vi "white line 1.vi"   [LabVIEW 2010, in "Line Follower.lvrbt"]
uses:
  Line Follower.lvrbt
  <vilib>/NXT/Block Support/NXT_InputPort.ctl
  <vilib>/NXT/Subs/MotorOutput.ctl
  <vilib>/NXT/Dual Mode Library/Sensors/Sonar_cm.vi
  <vilib>/NXT/Dual Mode Library/Sensors/Light_On.vi
  <vilib>/NXT/Dual Mode Library/Motors/MotorOn.vi
  <vilib>/NXT/Dual Mode Library/Motors/MotorBrake.vi
types:
  T1 = typedef "NXT_InputPort.ctl" = u8
  T2 = typedef "MotorOutput.ctl" = u8
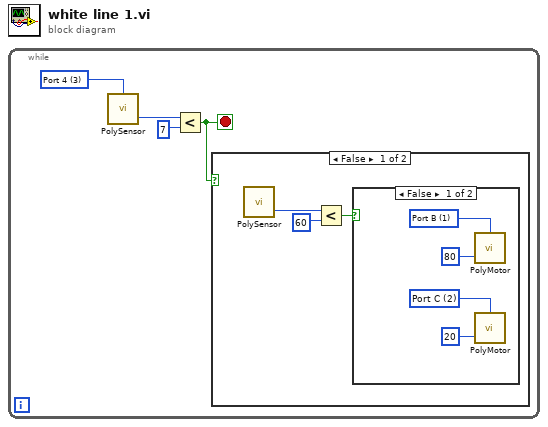
[diagram p0: block diagram]
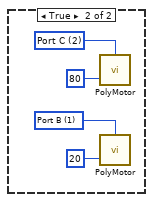
[diagram p2: hidden frame]
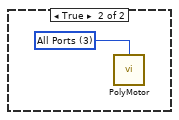
[diagram p3: hidden frame]
diagram:
  n1 = while {
    stop <- w2 stop-if-true
    w4 = T1 3 items=["Port 1", "Port 2", "Port 3", "Port 4"] ("Port (Port 4)")
    n2 = call-poly <vilib>:"PolySensor.vi"("Port (Port 4)"=w4) -> ("Distance (cm)"=w3:i16)  [unwired: 2 in, 1 out]
    n3 = Less?(x=w3, y=i16 7) -> (x < y?=w2:bool)
    n4 = case shown="False" w2 {
      frame False {
        n5 = call-poly <vilib>:"PolySensor.vi"() -> ("Scaled Value"=w7:i16)  [unwired: 3 in, 1 out]
        n6 = Less?(x=w7, y=i16 60) -> (x < y?=w6:bool)
        n7 = case shown="False" w6 {
          frame False {
            w10 = T2 2 items=["Port A"=0, "Port B"=1, "Port C"=2, "Ports A & B"=4, "Ports A & C"=5, "Ports B & C"=6, "All Ports"=3] ("Port (All Ports)")
            w8 = T2 1 items=["Port A"=0, "Port B"=1, "Port C"=2, "Ports A & B"=4, "Ports A & C"=5, "Ports B & C"=6, "All Ports"=3] ("Output Port (All Ports)")
            n8 = call-poly <vilib>:"PolyMotor.vi"("Power (75)"=80, "Output Port (All Ports)"=w8) -> ()  [unwired: 2 in, 1 out]
            n9 = call-poly <vilib>:"PolyMotor.vi"("Power (75)"=20, "Output Port (All Ports)"=w10) -> ()  [unwired: 2 in, 1 out]
          }
          frame True {
            w14 = T2 1 items=["Port A"=0, "Port B"=1, "Port C"=2, "Ports A & B"=4, "Ports A & C"=5, "Ports B & C"=6, "All Ports"=3] ("Port (All Ports)")
            w12 = T2 2 items=["Port A"=0, "Port B"=1, "Port C"=2, "Ports A & B"=4, "Ports A & C"=5, "Ports B & C"=6, "All Ports"=3] ("Output Port (All Ports)")
            n10 = call-poly <vilib>:"PolyMotor.vi"("Power (75)"=80, "Output Port (All Ports)"=w12) -> ()  [unwired: 2 in, 1 out]
            n11 = call-poly <vilib>:"PolyMotor.vi"("Power (75)"=20, "Output Port (All Ports)"=w14) -> ()  [unwired: 2 in, 1 out]
          }
        }
      }
      frame True {
        w16 = T2 3 items=["Port A"=0, "Port B"=1, "Port C"=2, "Ports A & B"=4, "Ports A & C"=5, "Ports B & C"=6, "All Ports"=3] ("Port (All Ports)")
        n12 = call-poly <vilib>:"PolyMotor.vi"("Port (All Ports)"=w16) -> ()  [unwired: 3 in, 1 out]
      }
    }
  }
